vi "hse-configuration_WriteDataDirectory.vi"(8 "error in (no error)":errorcluster, 10 "Data Directory":variant, 11 "hse-configuration in":refnum<class "hse-configuration.lvclass">) -> (0 "error out":errorcluster, 3 "hse-configuration out":refnum<class "hse-configuration.lvclass">)   [LabVIEW 2022 SP3, in "hse-configuration.lvclass"]
doc: "____\nHAMPEL SOFTWARE ENGINEERING v3.8.0 (2023-12-18 14:41)"
uses:
  hse-configuration.lvclass
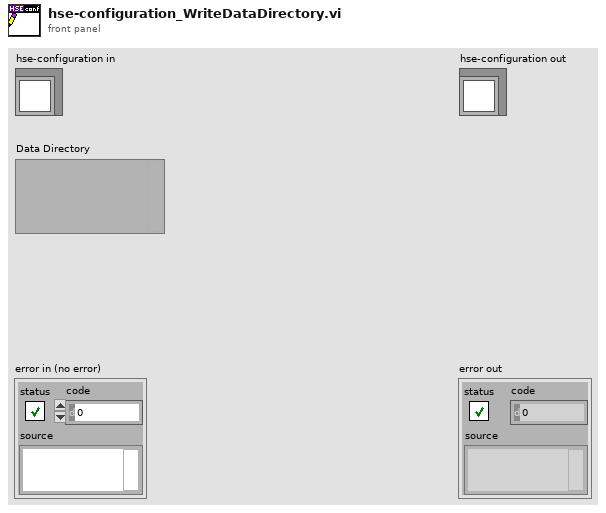
[diagram p1: front panel]
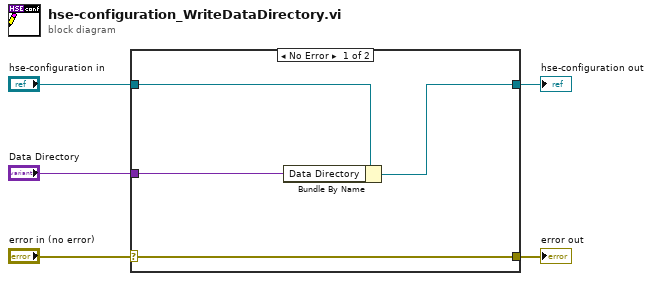
[diagram p0: block diagram]
diagram:
  n1 = case shown="No Error" "error in (no error)" {
    selector: "error in (no error)" -> [w9 w10]
    tunnel: [w9 w10] -> w4
    tunnel: [w7 w11] -> w2
    tunnel: "hse-configuration in" -> [w8 w11]
    tunnel: "Data Directory" -> [w6 _]
    frame No Error {
      n2 = Bundle By Name(cluster=w8, "Data Directory"=w6) -> (w7:refnum<class "hse-configuration.lvclass">)
    }
    frame Error {
    }
  }
  "error out" <- w4
  "hse-configuration out" <- w2
